vi "Report_Do.vi"(8 "error in (no error)":errorcluster, 9 "Results":T1[](array[typedef]), 10 "Project Builder in":refnum<class "Project Builder.lvclass">, 11 "Report Action in":refnum<class "Report Action.lvclass">) -> (0 "error out":errorcluster)   [LabVIEW 2020, in "ProjectBuilder.lvlib" / "Report Action.lvclass"]
uses:
  Report Action.lvclass
  Data/Report Data/Report Data.lvclass
  Action/Project Action/Project Action.lvclass
  Ctl/Ctl_Build Steps.ctl
  ProjectBuilder.lvlib
  Ctl/Ctl_Action Result.ctl
  Project Builder/Project Builder.lvclass
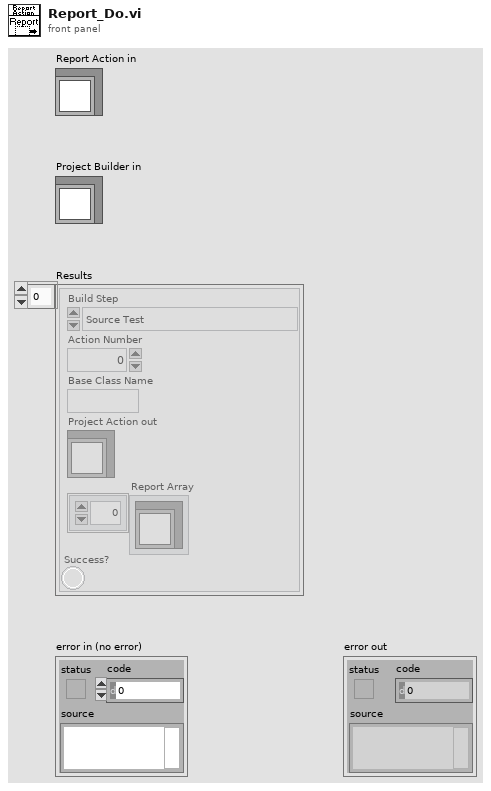
[diagram p1: front panel]
types:
  T1 = typedef "ProjectBuilder.lvlib/Ctl_Action Result.ctl" = cluster{"Build Step":T2, "Action Number":i32, "Base Class Name":string, "Project Action out":refnum<class "Project Action.lvclass">, "Report Array":refnum<class "Report Data.lvclass">[], "Success?":bool}
  T2 = typedef "ProjectBuilder.lvlib/Ctl_Build Steps.ctl" = enum16{"Source Test", "Build", "Post-Build Test", "Deploy", "Report"}
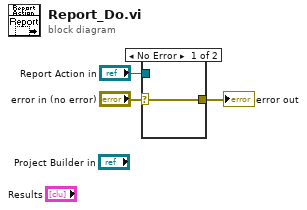
[diagram p0: block diagram]
diagram:
  n1 = case shown="No Error" "error in (no error)" {
    selector: "error in (no error)" -> [w4 w5]
    tunnel: [w4 w5] -> w2
    tunnel: "Report Action in" -> [_ _]
    frame No Error {
    }
    frame Error {
    }
  }
  "error out" <- w2
